vi "TCP_read.vi"(8 "error in (no error)":errorcluster, 10 "bytes to read":i32=10, 11 "TCP Network Connection in":refnum<k5>) -> (0 "error out":errorcluster, 2 "DataOut":string, 3 "TCP Network Connection out":refnum<k5>)   [LabVIEW 2019]
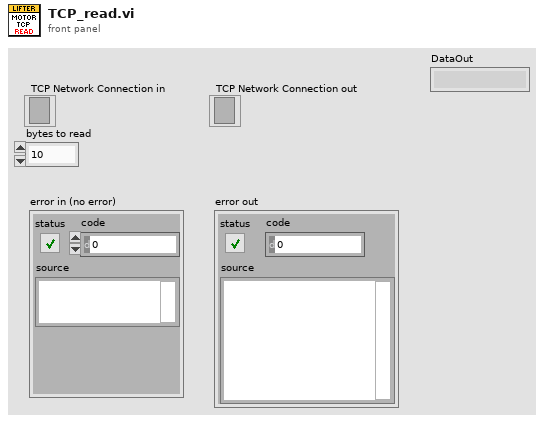
[diagram p1: front panel]
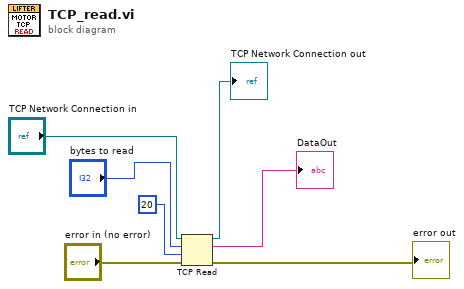
[diagram p0: block diagram]
diagram:
  n1 = TCP Read(connection ID="TCP Network Connection in", bytes to read="bytes to read", error in (no error)="error in (no error)", 9:20 ("timeout ms (25000)")) -> (connection ID out=→"TCP Network Connection out":refnum<k5>, data out=→"DataOut":string, error out=→"error out":errorcluster)  [unwired: 1 in]
